vi "Test.vi"() -> ()   [LabVIEW 2017]
panel:
  out "appended path":path
  out "Application Directory":path
  out "path 2":path
  out "path":path
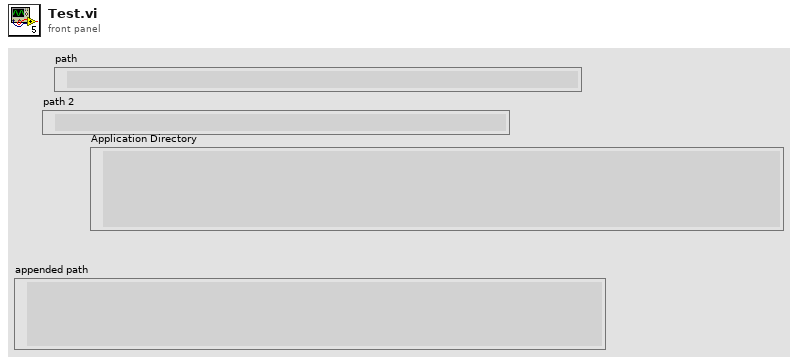
[diagram p1: front panel]
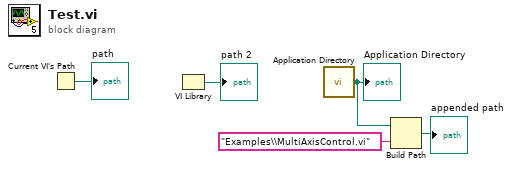
[diagram p0: block diagram]
diagram:
  n1 = Current VI's Path() -> (path=→"path":path)
  n2 = VI Library() -> (path=→"path 2":path)
  n3 = call <vilib>:"Application Directory.vi"() -> ("Application Directory"=w3:path)
  "Application Directory" <- w3
  n4 = Build Path(base path=w3, name or relative path="Examples\\MultiAxisControl.vi") -> (appended path=→"appended path":path)
